vi "Get Children Of Parent.vi"(8 "error in (no error)":errorcluster, 10 "Parent Tag":string, 11 "Tree Ref In":refnum<vi>) -> (0 "error out":errorcluster, 1 "Children Text":string[](array[string]), 2 "Children Tags":string[](array[string]), 3 "Tree Ref Out":refnum<vi>)   [LabVIEW 2011]
doc: "This VI will return all the <b>Children</b> tags under a <b>Parent Tag</b> of a tree that is passed in.\n-------------\nBrian Hoover (hooovahh)"
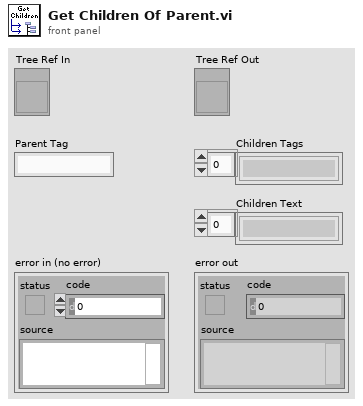
[diagram p1: front panel]
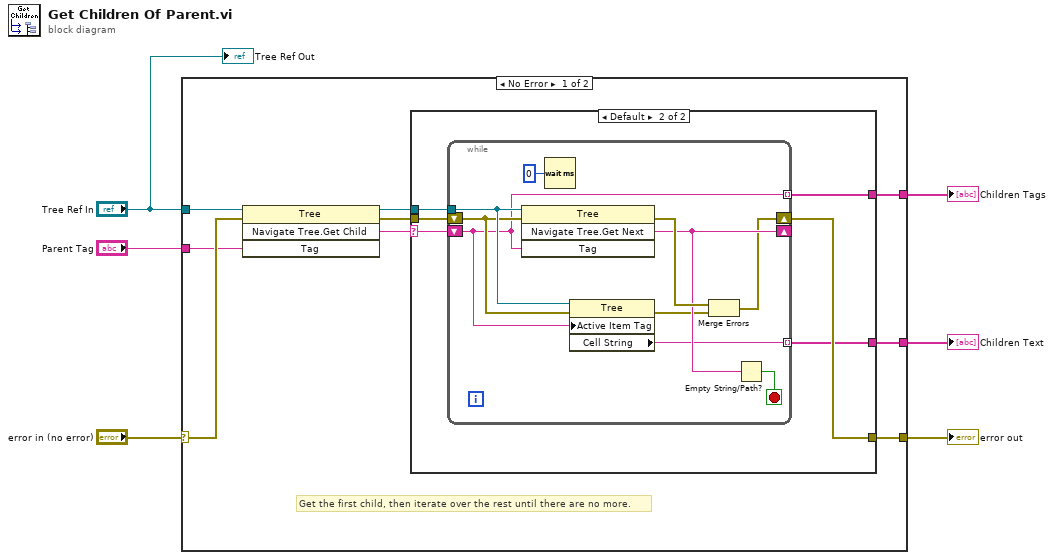
[diagram p0: block diagram]
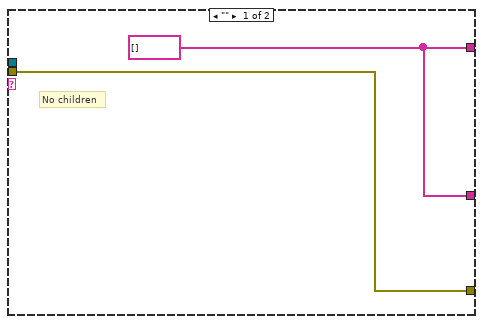
[diagram p2: hidden frame]
diagram:
  n1 = case shown="No Error" "error in (no error)" {
    selector: "error in (no error)" -> [w12 w34]
    tunnel: "Tree Ref In" -> [w15 _]
    tunnel: [w10 _] -> w4
    tunnel: [w9 w34] -> w5
    tunnel: "Parent Tag" -> [w8 _]
    tunnel: [w7 _] -> w1
    frame No Error {
      # "Get the first child, then iterate over the rest until there are no more."
      n2 = invoke class="Tree" method="Navigate Tree.Get Child"(reference=w15, error in=w12, "Tag"=w8) -> (reference out=w14:refnum<vi>, error out=w13:errorcluster, "Navigate Tree:Get Child"=w11:string)  [unwired: 1 in, 1 out]
      n3 = case shown="Default" w11 {
        selector: w11 -> [_ w18]
        tunnel: w14 -> [_ w23]
        tunnel: w13 -> [w17 w22]
        tunnel: [w16 w20] -> w10
        tunnel: [w17 w21] -> w9
        tunnel: [w16 w19] -> w7
        frame "" {
          w16 = string[] []
          # "No children"
        }
        frame Default {
          n4 = while {
            tunnel: w23 -> [w29]
            shift-right: [w25] -> w21
            shift-left: w22 -> [w28]
            shift-right: [w30] -> _
            shift-left: w18 -> [w27]
            tunnel: [w27] -> w20 mode=indexing
            tunnel: [w26] -> w19 mode=indexing
            stop <- w32 stop-if-true
            n5 = invoke class="Tree" method="Navigate Tree.Get Next"(reference=w29, error in=w28, "Tag"=w27) -> (error out=w33:errorcluster, "Navigate Tree:Get Next Item"=w30:string)  [unwired: 1 in, 2 out]
            n6 = Wait (ms)(milliseconds to wait=u32 0) -> ()  [unwired: 1 out]
            n7 = property class="Tree"(reference=w29, error in=w28, "Active Item Tag"=w27) -> (error out=w24:errorcluster, "Cell String"=w26:string)  [unwired: 1 out]
            n8 = Merge Errors(w33, w24) -> (w25:errorcluster)
            n9 = Empty String/Path?(string/path=w30) -> (empty?=w32:bool)
          }
        }
      }
    }
    frame Error {
    }
  }
  "error out" <- w5
  "Children Tags" <- w4
  "Children Text" <- w1
  "Tree Ref Out" <- "Tree Ref In"
